vi "Run.vi"(6 "Type Y":T2(ring), 7 "Type X":T2(ring), 8 "error in (no error)":errorcluster caption="entrée d'erreur (pas d'erreur)", 9 "Y":string[][](array[string]), 10 "X":string[][](array[string]), 11 "Argmin_min.lvclass":refnum<class "Argmin_min.lvclass">) -> (0 "error out":errorcluster caption="sortie d'erreur", 2 "Data":T1, 3 "Argmin_min.lvclass":refnum<class "Argmin_min.lvclass">)   [LabVIEW 2020, in "Argmin_min.lvclass"]
doc: "Returns : \n\n- argmin : numpy.ndarray\nY[argmin[i], :] is the row in Y that is closest to X[i, :].\n\n- distances : numpy.ndarray\ndistances[i] is the distance between the i-th row in X and the argmin[i]-th row in Y."
uses:
  Argmin_min.lvclass
  Argmin_min.lvclass/Argmin_min.ctl
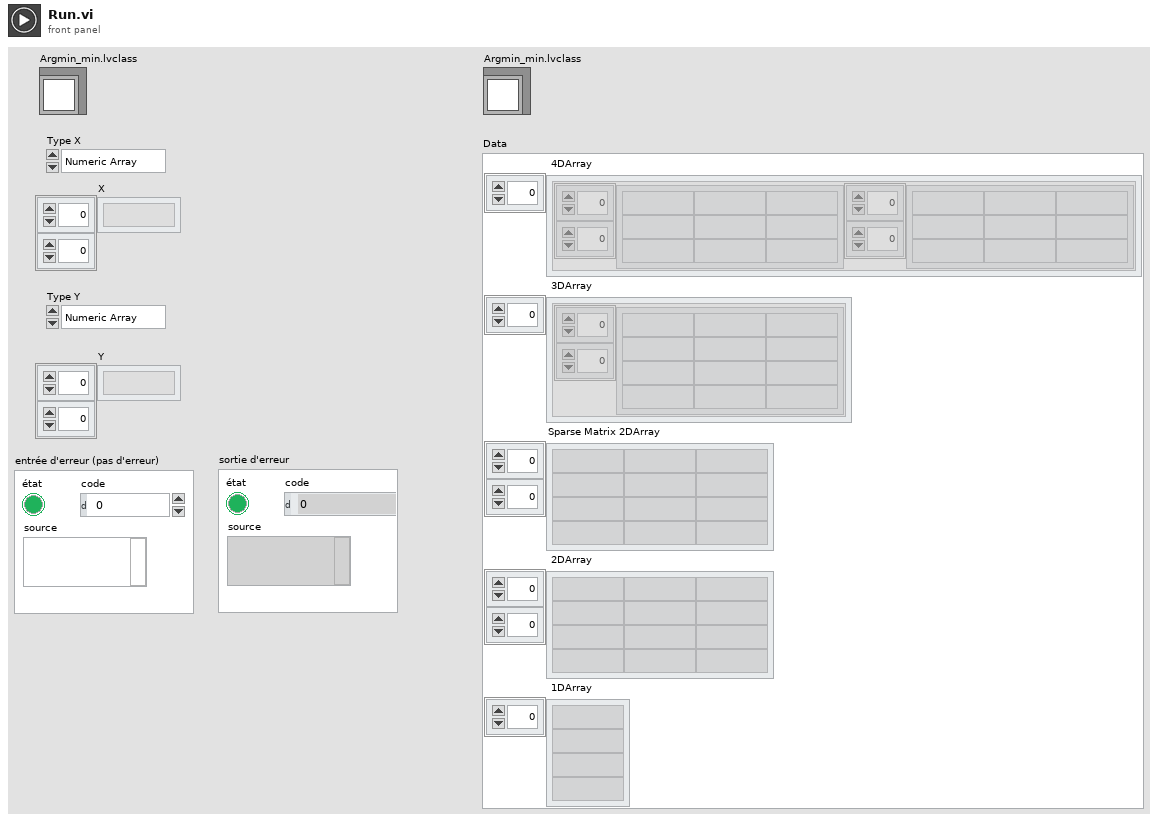
[diagram p1: front panel]
types:
  T1 = cluster{" 4DArray":cluster{"1":string[][], "2":string[][]}[], " 3DArray":cluster{"Tableau":string[][]}[], "Sparse Matrix 2DArray":string[][], " 2DArray":string[][], " 1DArray":string[]}
  T2 = enum16{"Numeric Array", "String Array", "Sparse"}
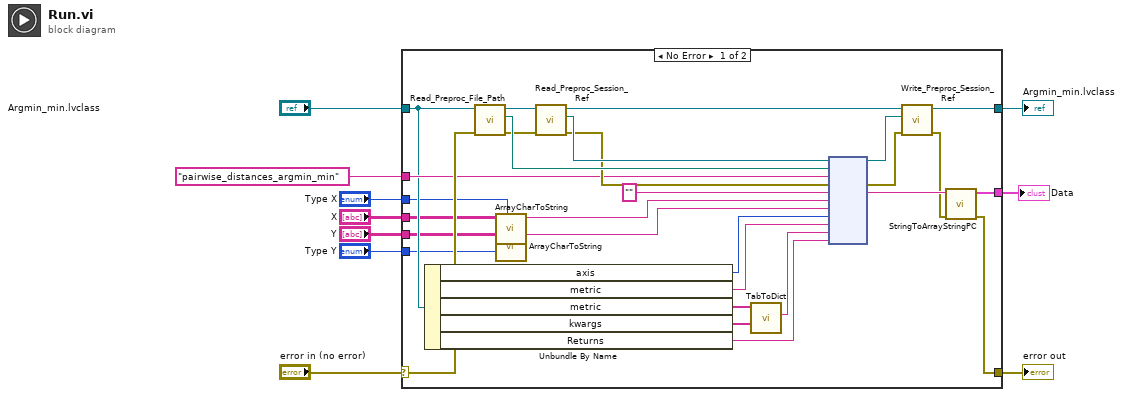
[diagram p0: block diagram]
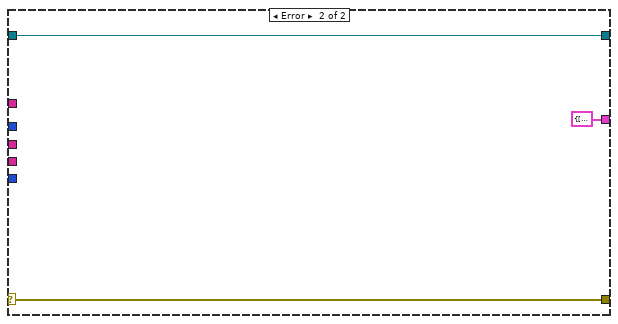
[diagram p2: hidden frame]
diagram:
  n1 = case shown="No Error" "error in (no error)" {
    selector: "error in (no error)" -> [w30 w42]
    tunnel: [w12 w42] -> w9
    tunnel: [w15 w41] -> w7
    tunnel: "Argmin_min.lvclass" -> [w28 w41]
    tunnel: "pairwise_distances_argmin_min" ("Fonction") -> [w29 _]
    tunnel: "X" -> [w21 _]
    tunnel: "Type X" -> [w20 _]
    tunnel: "Y" -> [w19 _]
    tunnel: "Type Y" -> [w18 _]
    tunnel: [w11 T1 {" 4DArray"=[], " 3DArray"=[], "Sparse Matrix 2DArray"=[], " 2DArray"=[], " 1DArray"=[]} ("Data")] -> w1
    frame No Error {
      n2 = Unbundle By Name(w28) -> ("axis"=w27:i32, "metric"=w26:string, "metric"=w25:string[], "kwargs"=w24:string[], "Returns"=w22:string)
      n3 = call-dynamic "Read_Preproc_File_Path.vi"("error in (no error)"=w30, "Python in"=w28) -> ("error out"=w34:errorcluster, "File_Path"=w37:path, "Python out"=w39:refnum<class "Argmin_min.lvclass">)  [unwired: 7 in]
      n4 = call "ArrayCharToString.vi"("Type"=w20, "TAB"=w21) -> ("Instruction"=w17:string)  [unwired: 9 in]
      n5 = call "ArrayCharToString.vi"("Type"=w18, "TAB"=w19) -> ("Instruction"=w16:string)  [unwired: 9 in]
      n6 = call-dynamic "Read_Preproc_Session_Ref.vi"("error in (no error)"=w34, "Python in"=w39) -> ("error out"=w35:errorcluster, "Session_ref"=w36:refnum<k35>, "Python out"=w38:refnum<class "Argmin_min.lvclass">)  [unwired: 7 in]
      n7 = call "TabToDict.vi"("String Value"=w24, "String key"=w25) -> ("Dict with string value"=w23:string)  [unwired: 8 in, 1 out]
      n8 = node(w36, w37, w29, w35, "", w17, w16, w27, w26, w23, w22) -> (w31:refnum<k35>, w33:errorcluster, w14:string)  [unwired: 6 in, 2 out]
      n9 = call-dynamic "Write_Preproc_Session_Ref.vi"("error in (no error)"=w33, "Session_ref"=w31, "Python in"=w38) -> ("error out"=w13:errorcluster, "Python out"=w15:refnum<class "Argmin_min.lvclass">)  [unwired: 7 in]
      n10 = call "StringToArrayStringPC.vi"("sortie d'erreur"=w13, "Return value"=w14) -> ("sortie d'erreur"=w12:errorcluster, "Data"=w11:T1)  [unwired: 8 in]
    }
    frame Error {
    }
  }
  "error out" <- w9
  "Argmin_min.lvclass" <- w7
  "Data" <- w1
